vi "read hdf calibration data.vi"(9 "sensor_comp":T1, 10 "case_id":string, 11 "file":string) -> (1 "sensor_comp out":T1, 2 "case_id out":string, 3 "file out":string, 5 "function return":i32)   [LabVIEW 2019, in "apdm.lvlib"]
doc: "APDM_EXPORT int apdm_read_hdf_calibration_data(char *file, char *case_id, apdm_sensor_compensation_t *sensor_comp);"
uses:
  apdm.lvlib
  Lee Lab/CP FES Walking 2018/Code/Working/LabVIEW/apdm.dll
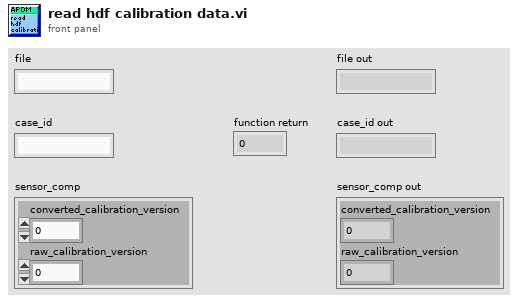
[diagram p1: front panel]
types:
  T1 = cluster{"converted_calibration_version":u32, "raw_calibration_version":u32}
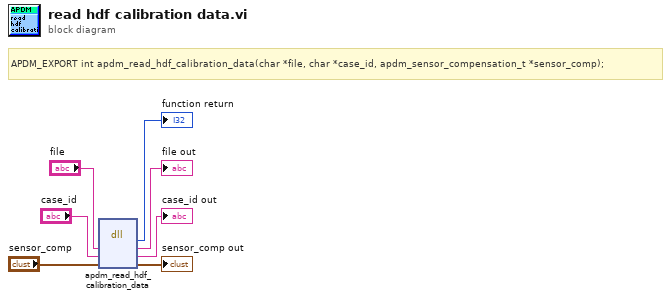
[diagram p0: block diagram]
diagram:
  # "APDM_EXPORT int apdm_read_hdf_calibration_data(char *file, char *case_id, apdm_sensor_compensation_t *sensor_comp);"
  n1 = dll-call lib="C:/Users/jfalesi/Dropbox/Lee Lab/CP FES Walking 2018/Code/Working/LabVIEW/apdm.*" fn="apdm_read_hdf_calibration_data"("file"="file", "case_id"="case_id", "sensor_comp"="sensor_comp") -> (→"function return":i32, "file"=→"file out":string, "case_id"=→"case_id out":string, "sensor_comp"=→"sensor_comp out":T1)  [unwired: 3 in, 2 out]
